vi "kalmanTimeUpdate.vi"(0 "Pk-1|k-1":T1, 1 "x_k-1|k-1":T1=[[0.0, 0.0, 0.0], [0.0, 0.0, 0.0], [0.0, 0.0, 0.0]], 2 "intervalo":dbl, 5 "error in (no error)":errorcluster) -> (14 "x_k|k out":T1, 16 "Pk|k out":T1, 19 "error out":errorcluster)   [LabVIEW 2023, in "Vision.lvclass"]
uses:
  Vision.lvclass
  <vilib>/Analysis/Matrix/Datatypes/RealMatrix.ctl
  <vilib>/Analysis/Matrix/Numeric/Multiply/Multiply - RM,RM.vi
  <vilib>/Analysis/Matrix/Numeric/Add/Add - RM,RM.vi
  <vilib>/Analysis/Matrix/NI_Matrix.lvlib
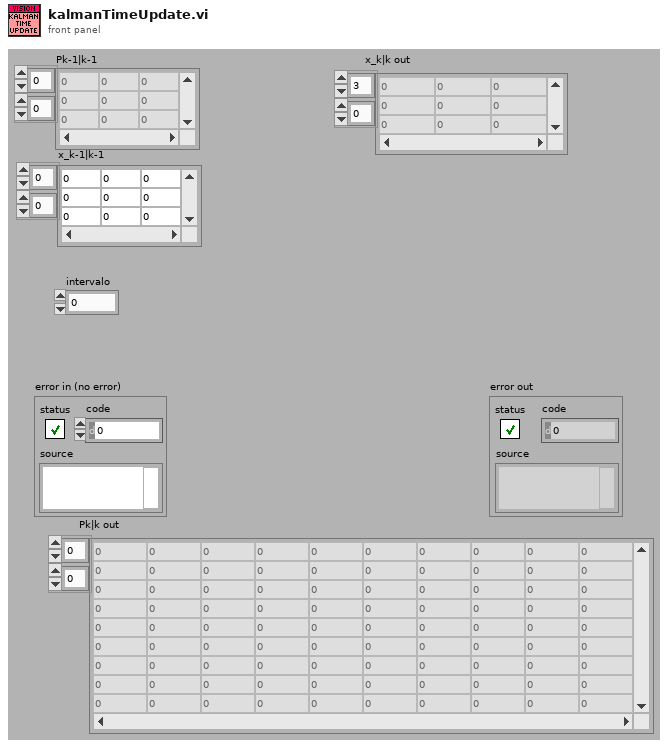
[diagram p1: front panel]
types:
  T1 = typedef "NI_Matrix.lvlib/RealMatrix.ctl" = dbl[][]
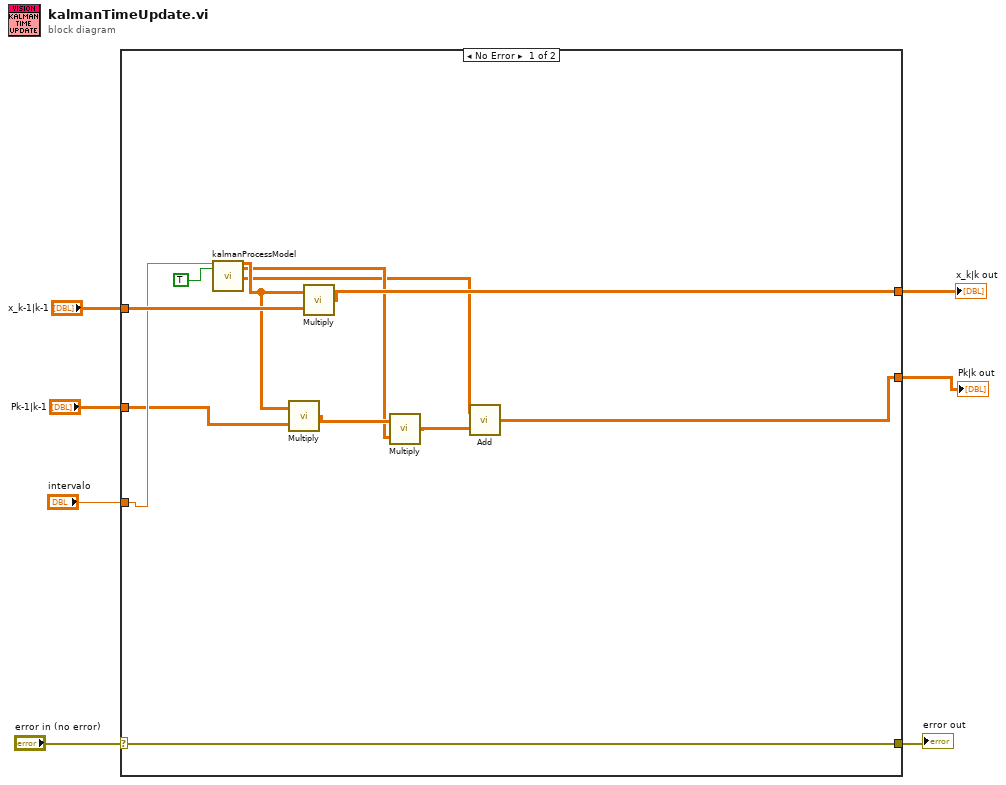
[diagram p0: block diagram]
diagram:
  n1 = case shown="No Error" "error in (no error)" {
    selector: "error in (no error)" -> [w19 w22]
    tunnel: [w19 w22] -> w6
    tunnel: "x_k-1|k-1" -> [w18 w21]
    tunnel: "Pk-1|k-1" -> [w13 w20]
    tunnel: [w17 w21] -> w3
    tunnel: [w8 w20] -> w2
    tunnel: "intervalo" -> [w15 _]
    frame No Error {
      n2 = call "kalmanProcessModel.vi"("intervalo"=w15, "Ball?"=TRUE) -> ("F"=w14:T1, "F'"=w11:T1, "Q"=w9:T1)  [unwired: 14 in, 1 out]
      n3 = call-poly <vilib>:"Multiply.vi"("Real Matrix B"=w13, "Real Matrix A"=w14) -> ("A * B"=w12:T1)
      n4 = call-poly <vilib>:"Multiply.vi"("Real Matrix B"=w18, "Real Matrix A"=w14) -> ("A * B"=w17:T1)
      n5 = call-poly <vilib>:"Multiply.vi"("Real Matrix B"=w11, "Real Matrix A"=w12) -> ("A * B"=w10:T1)
      n6 = call-poly <vilib>:"Add.vi"("Real Matrix B"=w10, "Real Matrix A"=w9) -> ("A + B"=w8:T1)
    }
    frame Error {
    }
  }
  "error out" <- w6
  "Pk|k out" <- w2
  "x_k|k out" <- w3
